vi "配方.vi"() -> (1 "起始行号":string[](array[string]), 2 "终止行号":string[](array[string]))   [LabVIEW 2018]
panel:
  out "end":i32[](array[numeric])
  out "start":i32[](array[numeric])
  out "数组 2":string[](array[string])=["A", "A", "B"]
  out "数值 3":i32
  out "数值 2":i32
  out "数组":string[](array[string])=["A", "B", "C"]
  out "数值":i32
  out "终止位置":string[](array[string])
  out "起始位置":string[](array[string])
  out "行号":string[](array[string])
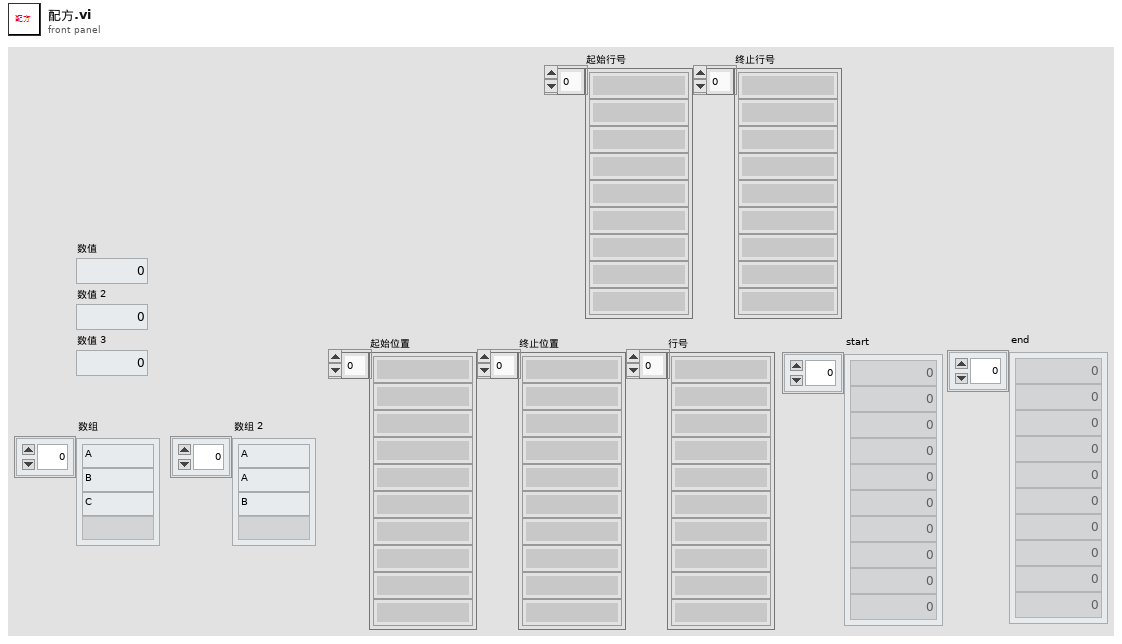
[diagram p1: front panel]
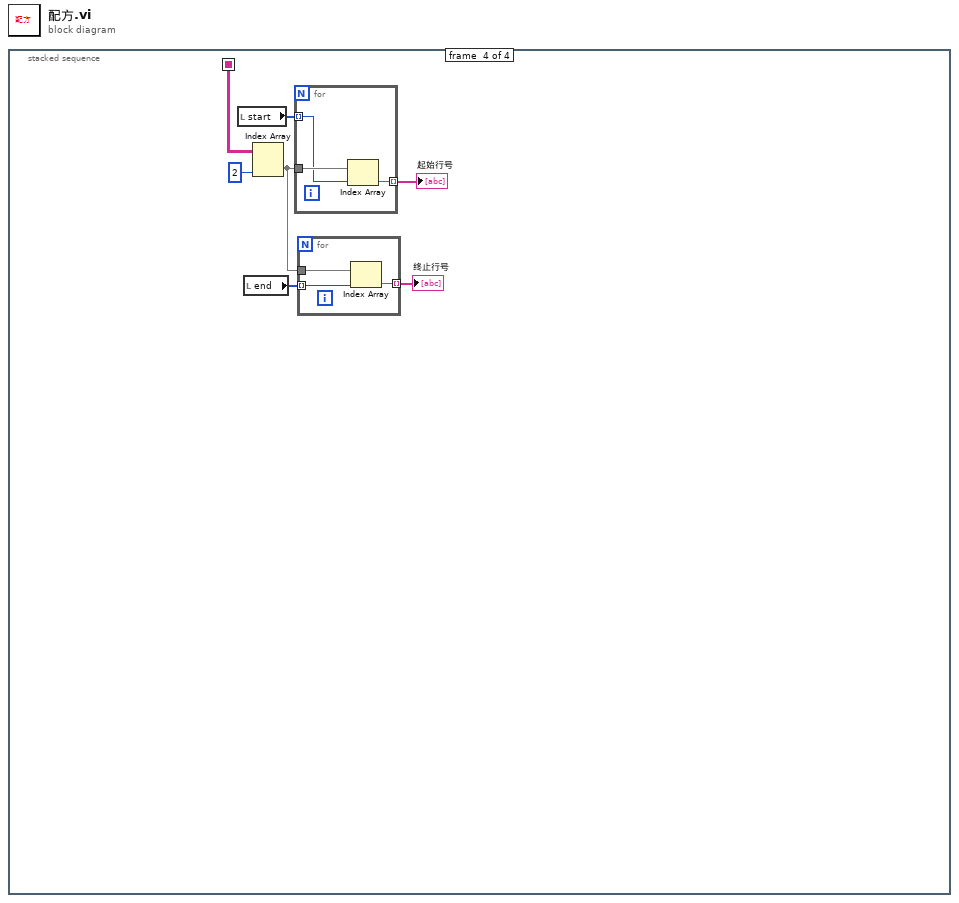
[diagram p0: block diagram]
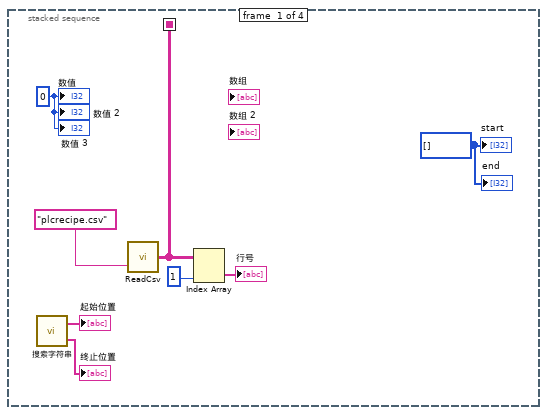
[diagram p2: hidden frame]
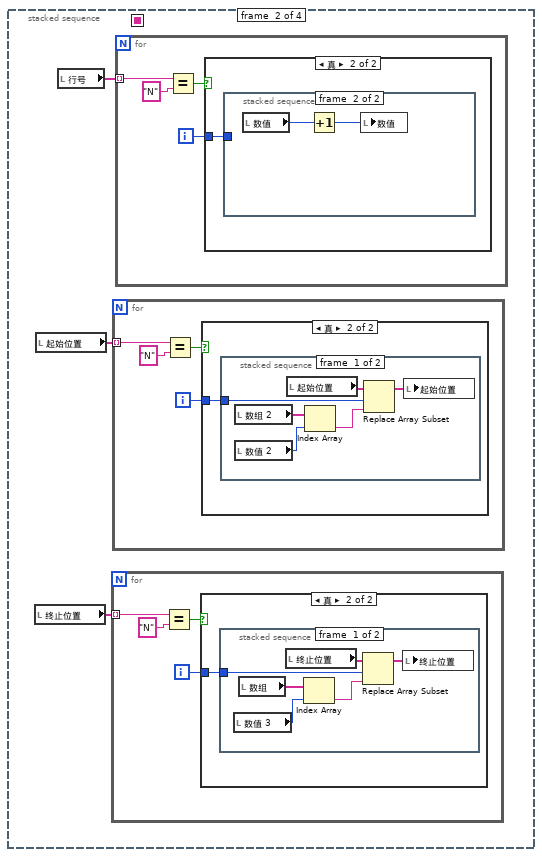
[diagram p3: hidden frame]
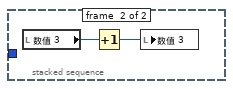
[diagram p5: hidden frame]
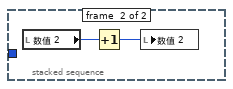
[diagram p7: hidden frame]
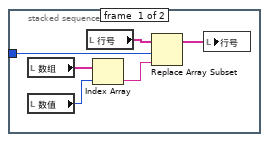
[diagram p9: hidden frame]
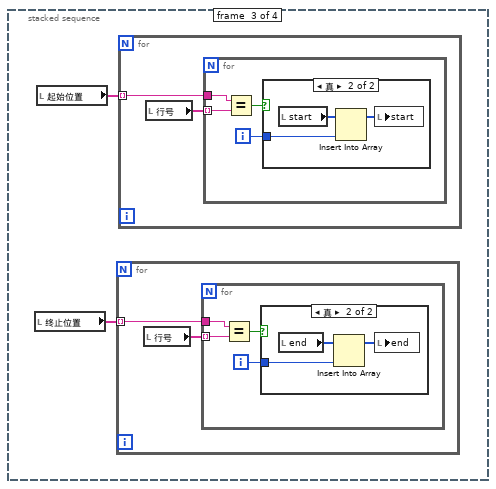
[diagram p10: hidden frame]
diagram:
  n1 = stacked-sequence {
    seq-local: [w1 _ _ _] -> [_ _ _ w77]
    frame #0 {
      w2 = i32[] [] ("tart")
      w3 = 0 ("数值")
      n2 = call "搜索字符串.vi"() -> ("起始位置"=→"起始位置":string[], "终止位置"=→"终止位置":string[])  [unwired: 1 in]
      n3 = call "ReadCsv.vi"("相对路径"="plcrecipe.csv") -> ("all rows"=w1:string[][])  [unwired: 1 in]
      n4 = Index Array(array=w1, index (col)=1 ("禁用的索引 (列)")) -> (element=→"行号":string[])  [unwired: 1 in]
      "数值" <- w3
      "数值 2" <- w3
      "数值 3" <- w3
      "end" <- w2
      "start" <- w2
    }
    frame #1 {
      n5 = local read "终止位置"() -> (w9:string[])
      n6 = local read "起始位置"() -> (w10:string[])
      n7 = local read "行号"() -> (w11:string[])
      n8 = for {
        tunnel: w9 -> [w15] mode=indexing
        i -> [w12]
        n9 = Equal?(x=w15, y="N") -> (x = y?=w13:bool)
        n10 = case shown="真" w13 {
          tunnel: w12 -> [_ w16]
          frame False {
          }
          frame True {
            n11 = stacked-sequence {
              tunnel: w16 -> [w17 _]
              frame #0 {
                n12 = local read "数值 3"() -> (w20:i32)
                n13 = local read "数组"() -> (w21:string[])
                n14 = local read "终止位置"() -> (w22:string[])
                n15 = Index Array(array=w21, index=w20) -> (element=w19:string)
                n16 = Replace Array Subset(array=w22, new element=w19, index=w17) -> (w18:string[])
                n17 = local write "终止位置"(w18) -> ()
              }
              frame #1 {
                n18 = local read "数值 3"() -> (w24:i32)
                n19 = Increment(x=w24) -> (x+1=w23:i32)
                n20 = local write "数值 3"(w23) -> ()
              }
            }
          }
        }
      }
      n21 = for {
        tunnel: w10 -> [w28] mode=indexing
        i -> [w25]
        n22 = Equal?(x=w28, y="N") -> (x = y?=w26:bool)
        n23 = case shown="真" w26 {
          tunnel: w25 -> [_ w29]
          frame False {
          }
          frame True {
            n24 = stacked-sequence {
              tunnel: w29 -> [w30 _]
              frame #0 {
                n25 = local read "数组 2"() -> (w34:string[])
                n26 = local read "数值 2"() -> (w33:i32)
                n27 = local read "起始位置"() -> (w35:string[])
                n28 = Index Array(array=w34, index=w33) -> (element=w32:string)
                n29 = Replace Array Subset(array=w35, new element=w32, index=w30) -> (w31:string[])
                n30 = local write "起始位置"(w31) -> ()
              }
              frame #1 {
                n31 = local read "数值 2"() -> (w37:i32)
                n32 = Increment(x=w37) -> (x+1=w36:i32)
                n33 = local write "数值 2"(w36) -> ()
              }
            }
          }
        }
      }
      n34 = for {
        tunnel: w11 -> [w41] mode=indexing
        i -> [w38]
        n35 = Equal?(x=w41, y="N") -> (x = y?=w39:bool)
        n36 = case shown="真" w39 {
          tunnel: w38 -> [_ w42]
          frame False {
          }
          frame True {
            n37 = stacked-sequence {
              tunnel: w42 -> [w43 _]
              frame #0 {
                n38 = local read "数组"() -> (w47:string[])
                n39 = local read "数值"() -> (w46:i32)
                n40 = local read "行号"() -> (w48:string[])
                n41 = Index Array(array=w47, index=w46) -> (element=w45:string)
                n42 = Replace Array Subset(array=w48, new element=w45, index=w43) -> (w44:string[])
                n43 = local write "行号"(w44) -> ()
              }
              frame #1 {
                n44 = local read "数值"() -> (w50:i32)
                n45 = Increment(x=w50) -> (x+1=w49:i32)
                n46 = local write "数值"(w49) -> ()
              }
            }
          }
        }
      }
    }
    frame #2 {
      n47 = local read "终止位置"() -> (w51:string[])
      n48 = local read "起始位置"() -> (w52:string[])
      n49 = for {
        tunnel: w51 -> [w53] mode=indexing
        n50 = local read "行号"() -> (w54:string[])
        n51 = for {
          tunnel: w54 -> [w58] mode=indexing
          tunnel: w53 -> [w57]
          i -> [w55]
          n52 = Equal?(x=w57, y=w58) -> (x = y?=w56:bool)
          n53 = case shown="真" w56 {
            tunnel: w55 -> [_ w60]
            frame False {
            }
            frame True {
              n54 = local read "end"() -> (w61:i32[])
              n55 = Insert Into Array(array=w61, new element=w60) -> (w59:i32[])  [unwired: 1 in]
              n56 = local write "end"(w59) -> ()
            }
          }
        }
      }
      n57 = for {
        tunnel: w52 -> [w62] mode=indexing
        n58 = local read "行号"() -> (w63:string[])
        n59 = for {
          tunnel: w63 -> [w67] mode=indexing
          tunnel: w62 -> [w66]
          i -> [w64]
          n60 = Equal?(x=w66, y=w67) -> (x = y?=w65:bool)
          n61 = case shown="真" w65 {
            tunnel: w64 -> [_ w69]
            frame False {
            }
            frame True {
              n62 = local read "start"() -> (w70:i32[])
              n63 = Insert Into Array(array=w70, new element=w69) -> (w68:i32[])  [unwired: 1 in]
              n64 = local write "start"(w68) -> ()
            }
          }
        }
      }
    }
    frame #3 {
      n65 = local read "start"() -> (w75:i32[])
      n66 = local read "end"() -> (w72:i32[])
      n67 = Index Array(array=w77, index (col)=2 ("禁用的索引 (列)")) -> (element=w73:string[])  [unwired: 1 in]
      n68 = for {
        tunnel: w73 -> [w83]
        tunnel: w75 -> [w81] mode=indexing
        tunnel: [w82] -> w74 mode=indexing
        n69 = Index Array(array=w83, index=w81) -> (element=w82:string)
      }
      "起始行号" <- w74
      n70 = for {
        tunnel: w73 -> [w80]
        tunnel: [w79] -> w71 mode=indexing
        tunnel: w72 -> [w78] mode=indexing
        n71 = Index Array(array=w80, index=w78) -> (element=w79:string)
      }
      "终止行号" <- w71
    }
  }
